vi "Initialize Memory Injection Waveform Voltage.vi"() -> (0 "Init Data Out":fxp<+/-,24,5>[](array[numeric]))   [LabVIEW 2015]
panel:
  out "Waveform Graph":dbl[](graph)
  # "For Initialization VI requirements and help, please read directions located on Block Diagram."
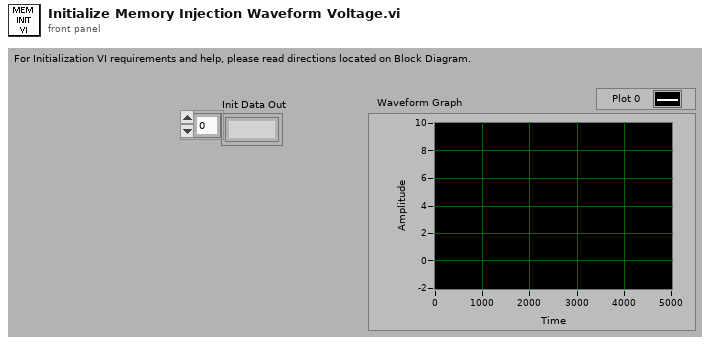
[diagram p1: front panel]
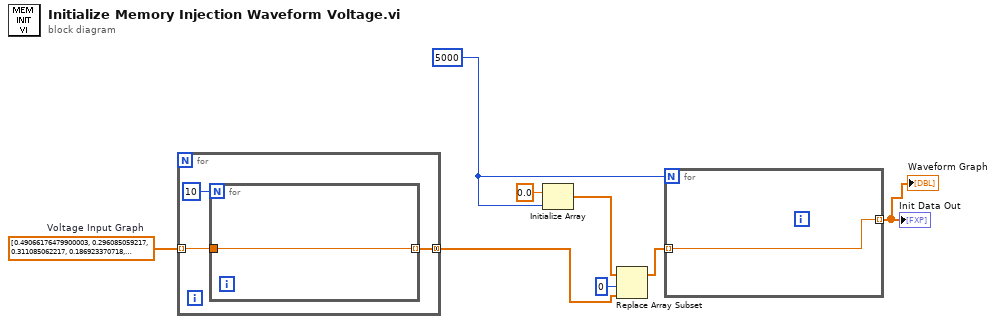
[diagram p0: block diagram]
diagram:
  w8 = dbl[] [0.49066176479900003, 0.296085059217, 0.311085062217, 0.186923370718, 0.296085059217, 0.311085062217, 0.186923370718, 0.0915095183019, 0.0894263512186, 0.288168390967, 0.19400503880099998, 0.200255040051, 0.0852598503853, -0.11473252294649999, -0.0205695041139, 8.42951835257, 8.61618505657, 8.50785170157, 8.19911830649, -0.11473252294649999, -0.0205695041139, 4.01428413619, 3.8809507761899997, -0.0205695041139, 3.8959507791899997, -0.11473252294649999, 0.0894263512186, 3.8959507791899997, 3.77011742069, -0.0205695041139, 3.8959507791899997, 3.65970073194, -0.455136757694, -0.1176490235298, -0.11473252294649999, 3.74803408294, -0.626796792026, -0.011403168947299999, -0.239311714529, -0.218895043779, -0.11473252294649999, 3.22221731111, -0.218895043779, 1.5202053040410002, -0.0205695041139, 3.8959507791899997, -0.218478377029, 3.74803408294, -0.1176490235298, 3.77011742069, -0.1301486926964, -0.1176490235298, -0.11473252294649999, -0.1301486926964, 4.133017493270001, -0.11473252294649999, 4.06718414677, -0.218895043779, -0.011403168947299999, -0.1301486926964, -0.218895043779, 3.8809507761899997, -0.1301486926964, 4.01428413619, -0.011403168947299999, -0.1301486926964, 3.77845075569, -0.11473252294649999, 3.85386743744, -0.1176490235298, -0.323058397945, -0.0205695041139, -0.320558397445, 3.99220079844, -0.0205695041139, 4.01428413619, -0.11473252294649999, 0.200255040051, -0.218895043779, -0.218478377029, 4.6046675876, 0.0852598503853, 3.8809507761899997, -0.1301486926964, 4.01428413619, -0.218478377029, -0.239311714529, -0.218895043779, -0.11473252294649999, 3.85386743744, -0.1176490235298, 3.77011742069, -0.1301486926964, -0.320558397445, 3.65970073194, -0.0205695041139, 4.133017493270001, -0.218478377029, 4.06718414677, -0.01598631986393, 0.19400503880099998, -0.0205695041139, -0.01598631986393, 3.54930070986, -0.1301486926964, 4.01428413619, -0.11473252294649999, -0.455136757694, -0.218895043779, -0.218478377029, 3.74803408294, -0.218895043779, 4.10343415402, -0.1301486926964, -0.218895043779, -0.011403168947299999, -0.1301486926964, 3.77845075569, -0.218478377029, 4.06718414677, -0.218895043779, 0.0915095183019, 0.0894263512186, 0.49066176479900003, 0.398165079633, 0.311085062217, 0.0852598503853, 0.19400503880099998, 0.200255040051, 0.389415077883]  # Voltage Input Graph
  w7 = 5000 ("Number of Elements")
  n1 = for {
    tunnel: [w11] -> w2 mode=concatenating
    tunnel: w8 -> [w10] mode=indexing
    n2 = for {
      N: 10 -> [_]
      tunnel: [w12] -> w11 mode=indexing
      tunnel: w10 -> [w12]
    }
  }
  n3 = Initialize Array(0.0 ("element"), w7) -> (w5:dbl[])
  n4 = Replace Array Subset(array=w5, new element=w2, index=0) -> (w3:dbl[])
  n5 = for {
    N: w7 -> [_]
    tunnel: [w13] -> w1 mode=indexing
    tunnel: w3 -> [w13] mode=indexing
  }
  "Init Data Out" <- w1
  "Waveform Graph" <- w1
